vi "Get Gamma Parameter Info.vi"(8 "error in (no error)":errorcluster, 11 "Stream":refnum<data-value>) -> (0 "error out":errorcluster, 2 "Info":T1, 3 "Stream (duplicate)":refnum<data-value>)   [LabVIEW 2020, in "g_ar_toolkit.capture.lvlib" / "CameraStream.lvclass"]
uses:
  CameraStream.lvclass
  CameraStream.lvclass/CameraStream.ctl
  Camera Parameters.ctl
  Camera Parameter Information.ctl
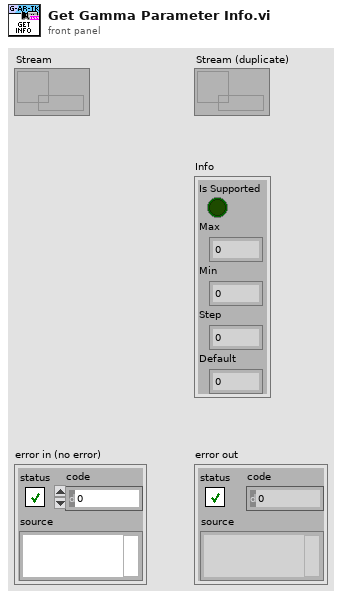
[diagram p1: front panel]
types:
  T1 = typedef "g_ar_toolkit.capture.lvlib/CameraStream.lvclass/Camera Parameter Information.ctl" = cluster{"Is Supported":bool, "Max":i32, "Min":i32, "Step":i32, "Default":i32}
  T2 = typedef "g_ar_toolkit.capture.lvlib/CameraStream.lvclass/Camera Parameters.ctl" = enum8{"EXPOSURE_ABSOLUTE", "FOCUS_ABSOLUTE", "ZOOM_ABSOLUTE", "WHITE_BALANCE_TEMPERATURE", "BRIGHTNESS", "CONTRAST", "SATURATION", "GAMMA", "HUE", "SHARPNESS", "BACKLIGHT_COMPENSATION", "POWER_LINE_FREQUENCY"}
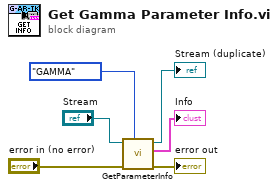
[diagram p0: block diagram]
diagram:
  n1 = call "GetParameterInfo.vi"("Camera Parameter"=Camera_Parameters."GAMMA", "error in (no error)"="error in (no error)", "Stream"="Stream") -> ("error out"=→"error out":errorcluster, "Info"=→"Info":T1, "Stream (duplicate)"=→"Stream (duplicate)":refnum<data-value>)  [unwired: 6 in]
